vi "Periodic Tasks.vi"(8 "error in":errorcluster) -> ()   [LabVIEW 2019]
doc: "This VI runs in parallel to other tasks. It can contain as many user-defined periodic loops as you need. These can carry out PID or other sorts of timed response."
uses:
  <vilib>/Rock Robotics/WPI/DriverStation/WPI_DriverStationRobotMode2.ctl
  <vilib>/Rock Robotics/WPI/Utilities/WPI_GetSetVariantRefNum.vi
  Robot Global Data.vi
  <vilib>/Rock Robotics/Network Tables/NT Write Boolean.vi
  <vilib>/Rock Robotics/Network Tables/NT Write Number.vi
  <vilib>/Rock Robotics/WPI/RobotDrive/WPI_RobotDriveArcadeDrive_Standard(NoSaturation).vi
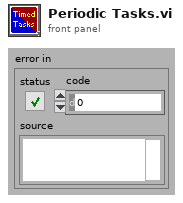
[diagram p1: front panel]
types:
  T1 = typedef "WPI_JoystickDevRef.ctl" = cluster{"Device":T2}
  T2 = typedef "WPI_JoystickDeviceEnum.ctl" = enum16{"USB 0", "USB 1", "USB 2", "USB 3", "USB 4", "USB 5"}
  T3 = typedef "WPI_RobotDriveDevRef.ctl" = cluster{"DevStatus":errorcluster, "Motors[]":T4[], "Square Inputs":bool, "Max Output":dbl}
  T4 = typedef "WPI_MotorControlDeviceRef.ctl" = cluster{"DeviceStatus":errorcluster, "Type":T5, "PWM":cluster{"PWM Channel":T6, "DeadBand":T7}, "CAN":cluster{"Device Number":u8, "SetOutput VI Ref":variant, "GetOutput VI Ref":variant, "Enable VI Ref":variant, "Disable VI Ref":variant, "Data":variant}, "Invert":bool, "DIO PWM":cluster{"PWM \"Enable\" Channel":T6, "DIOChannel":T8, "PWM Rate":dbl}}
  T5 = typedef "WPI_MotorControlType.ctl" = enum16{"PWM", "CAN", "DIO PWM"}
  T6 = typedef "FPGA_DIOPWMChannel.ctl" = enum8{"PWM 0", "PWM 1", "PWM 2", "PWM 3", "PWM 4", "PWM 5", "PWM 6", "PWM 7", "PWM 8", "PWM 9", "PWM MXP 0", "PWM MXP 1", "PWM MXP 2", "PWM MXP 3", "PWM MXP 4", "PWM MXP 5", "PWM MXP 6", "PWM MXP 7", "PWM MXP 8", "PWM MXP 9", "Invalid"}
  T7 = typedef "WPI_PWMDeadband.ctl" = cluster{"Name":string, "maxPositivePwm":i32, "minPositivePwm":i32, "centerPwm":i32, "maxNegativePwm":i32, "minNegativePwm":i32, "angularRange":u16}
  T8 = typedef "FPGA_DIOChannel.ctl" = enum8{"DIO 0", "DIO 1", "DIO 2", "DIO 3", "DIO 4", "DIO 5", "DIO 6", "DIO 7", "DIO 8", "DIO 9", "DIO MXP 0", "DIO MXP 1", "DIO MXP 2", "DIO MXP 3", "DIO MXP 4", "DIO MXP 5", "DIO MXP 6", "DIO MXP 7", "DIO MXP 8", "DIO MXP 9", "DIO MXP 10", "DIO MXP 11", "DIO MXP 12", "DIO MXP 13", "DIO MXP 14", "DIO MXP 15", "SPI Port CS1", "SPI Port CS2", "SPI Port CS3", "SPI Port MISO", "SPI Port MOSI", "Invalid"}
  T9 = cluster{"JoystickDevRef":T1, "RobotDriveDevRef":T3}
  T10 = typedef "WPI_DriverStationRobotMode2.ctl" = enum16{"Autonomous Disabled", "Autonomous Enabled", "Teleop Disabled", "Teleop Enabled", "Disconnected", "Finish", "Test Disabled", "Test Enabled", "Emergency Stopped"}
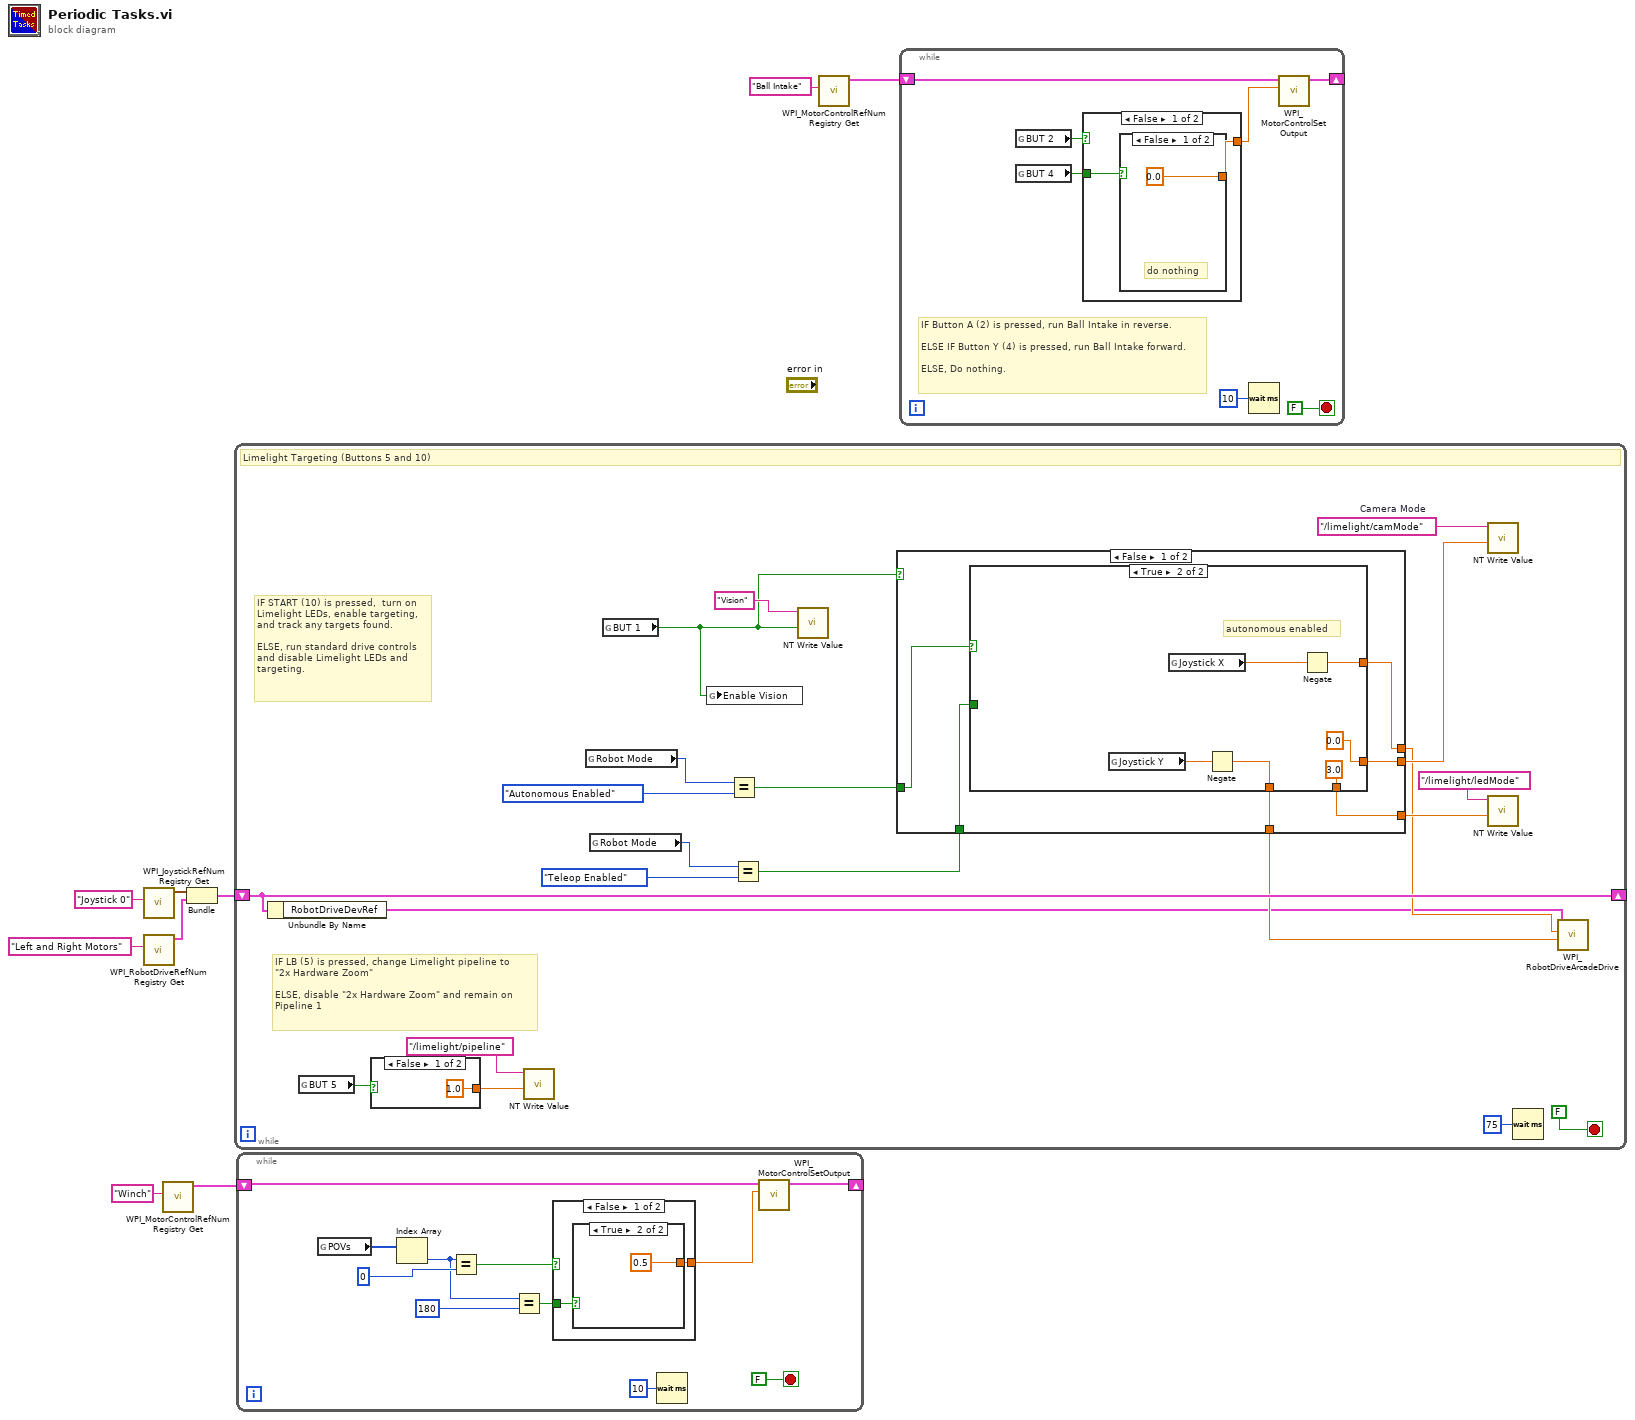
[diagram p0: block diagram]
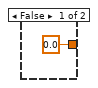
[diagram p2: hidden frame]
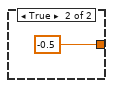
[diagram p3: hidden frame]
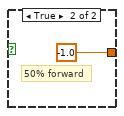
[diagram p4: hidden frame]
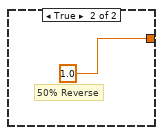
[diagram p5: hidden frame]
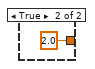
[diagram p6: hidden frame]
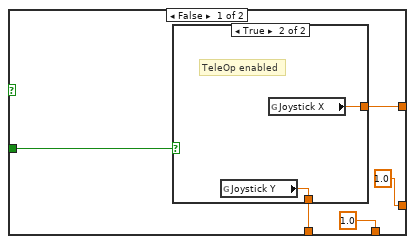
[diagram p7: hidden frame]
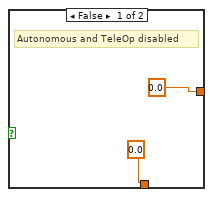
[diagram p8: hidden frame]
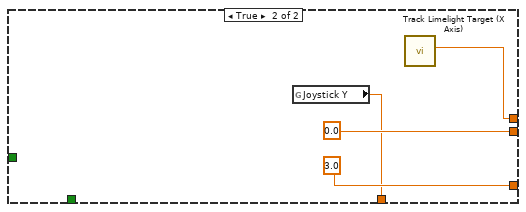
[diagram p9: hidden frame]
diagram:
  n1 = call <vilib>:"WPI_JoystickRefNum Registry Get.vi"("refnum name"="Joystick 0") -> ("JoystickDevRef"=w7:T1)  [unwired: 1 in, 9 out]
  n2 = call <vilib>:"WPI_RobotDriveRefNum Registry Get.vi"("refnum name"="Left and Right Motors") -> ("RobotDriveDevRef"=w6:T3)  [unwired: 1 in, 9 out]
  n3 = call <vilib>:"WPI_MotorControlRefNum Registry Get.vi"("refnum name"="Winch") -> ("MotorControlDevRef"=w2:T4)  [unwired: 9 in, 1 out]
  n4 = Bundle("JoystickDevRef"=w7, "RobotDriveDevRef"=w6) -> (w5:T9)  [unwired: 1 out]
  n5 = while {
    shift-right: [w29] -> _
    shift-left: w5 -> [w29]
    stop <- FALSE stop-if-true
    w27 = "/limelight/camMode"  # Camera Mode
    # "IF LB (5) is pressed, change Limelight pipeline to \n\"2x Hardware Zoom\"\n\nELSE, disable \"2x Hardware Zoom\" and remain on\nPipeline 1"
    # "IF START (10) is pressed,  turn on\nLimelight LEDs, enable targeting,\nand track any targets found.\n\nELSE, run standard drive controls\nand disable Limelight LEDs and \ntargeting."
    # "Limelight Targeting (Buttons 5 and 10)"
    n6 = Unbundle By Name(w29) -> ("RobotDriveDevRef"=w19:T3)
    n7 = global read "Robot Global Data.vi" "BUT 5"() -> (w11:bool)
    n8 = case shown="False" w11 {
      tunnel: [1.0 ("Numeric") 2.0 ("Numeric")] -> w12
      frame False {
      }
      frame True {
      }
    }
    n9 = call-poly <vilib>:"NT Write Value.vi"("Numeric"=w12, "Name"="/limelight/pipeline") -> ()  [unwired: 9 in, 1 out]
    n10 = global read "Robot Global Data.vi" "Robot Mode"() -> (w18:T10)
    n11 = global read "Robot Global Data.vi" "Robot Mode"() -> (w14:T10)
    n12 = global read "Robot Global Data.vi" "BUT 1"() -> (w10:bool)
    n13 = global write "Robot Global Data.vi" "Enable Vision"(w10) -> ()
    n14 = Equal?(x=w18, y=WPI_DriverStationRobotMode2."Autonomous Enabled") -> (x = y?=w16:bool)
    n15 = Equal?(x=w14, y=WPI_DriverStationRobotMode2."Teleop Enabled") -> (x = y?=w13:bool)
    n16 = call-poly <vilib>:"NT Write Value.vi"("Boolean"=w10, "Name"="Vision") -> ()  [unwired: 9 in, 1 out]
    n17 = case shown="False" w10 {
      tunnel: [w34 0.0 ("Numeric")] -> w26
      tunnel: [w33 3.0 ("Numeric")] -> w25
      tunnel: [w37 w55] -> w20
      tunnel: [w38 w54] -> w21
      tunnel: w16 -> [w35 _]
      tunnel: w13 -> [w36 _]
      frame False {
        n18 = case shown="True" w35 {
          tunnel: [w42 w52] -> w38
          tunnel: [w43 w51] -> w37
          tunnel: w36 -> [w41 _]
          tunnel: [1.0 ("Numeric") 0.0 ("Numeric")] -> w34
          tunnel: [1.0 ("Numeric") 3.0 ("Numeric")] -> w33
          frame False {
            n19 = case shown="True" w41 {
              tunnel: [0.0 ("Joystick X") w47] -> w43
              tunnel: [0.0 ("Joystick Y") w46] -> w42
              frame False {
                # "Autonomous and TeleOp disabled"
              }
              frame True {
                # "TeleOp enabled"
                n20 = global read "Robot Global Data.vi" "Joystick Y"() -> (w46:dbl)
                n21 = global read "Robot Global Data.vi" "Joystick X"() -> (w47:dbl)
              }
            }
          }
          frame True {
            # "autonomous enabled"
            n22 = global read "Robot Global Data.vi" "Joystick Y"() -> (w53:dbl)
            n23 = global read "Robot Global Data.vi" "Joystick X"() -> (w50:dbl)
            n24 = Negate(x=w53) -> (-x=w52:dbl)
            n25 = Negate(x=w50) -> (-x=w51:dbl)
          }
        }
      }
      frame True {
        n26 = global read "Robot Global Data.vi" "Joystick Y"() -> (w54:dbl)
        n27 = call "Track Limelight Target (X Axis).vi"() -> ("Joystick X"=w55:dbl)  [unwired: 11 in]
      }
    }
    n28 = call-poly <vilib>:"NT Write Value.vi"("Numeric"=w26, "Name"=w27) -> ()  [unwired: 9 in, 1 out]
    n29 = call-poly <vilib>:"NT Write Value.vi"("Numeric"=w25, "Name"="/limelight/ledMode" ("LED Mode")) -> ()  [unwired: 9 in, 1 out]
    n30 = Wait (ms)(milliseconds to wait=u32 75) -> ()  [unwired: 1 out]
    n31 = call-poly <vilib>:"WPI_RobotDriveArcadeDrive.vi"("Y axis value"=w21, "X axis value"=w20, "RobotDriveDevRef"=w19) -> ()  [unwired: 6 in, 3 out]
  }
  n32 = while {
    shift-right: [w67] -> _
    shift-left: w2 -> [w66]
    stop <- FALSE stop-if-true
    n33 = global read "Robot Global Data.vi" "POVs"() -> (w64:i16[])
    n34 = Index Array(array=w64) -> (element=w60:i16)  [unwired: 1 in]
    n35 = Equal?(x=w60, y=i16 0) -> (x = y?=w63:bool)
    n36 = Equal?(x=w60, y=i16 180) -> (x = y?=w61:bool)
    n37 = case shown="False" w63 {
      tunnel: [w70 -0.5 ("Output")] -> w65
      tunnel: w61 -> [w69 _]
      frame False {
        n38 = case shown="True" w69 {
          tunnel: [0.0 ("Output") 0.5 ("Output")] -> w70
          frame False {
          }
          frame True {
          }
        }
      }
      frame True {
      }
    }
    n39 = Wait (ms)(milliseconds to wait=u32 10) -> ()  [unwired: 1 out]
    n40 = call <vilib>:"WPI_MotorControlSetOutput.vi"("Output"=w65, "MotorControlDevRef"=w66) -> ("MotorControlDevRef"=w67:T4)  [unwired: 7 in, 2 out]
  }
  n41 = call <vilib>:"WPI_MotorControlRefNum Registry Get.vi"("refnum name"="Ball Intake") -> ("MotorControlDevRef"=w3:T4)  [unwired: 9 in, 1 out]
  n42 = while {
    shift-right: [w77] -> _
    shift-left: w3 -> [w78]
    stop <- FALSE stop-if-true
    # "IF Button A (2) is pressed, run Ball Intake in reverse. \n\nELSE IF Button Y (4) is pressed, run Ball Intake forward.\n\nELSE, Do nothing."
    n43 = global read "Robot Global Data.vi" "BUT 2"() -> (w75:bool)
    n44 = global read "Robot Global Data.vi" "BUT 4"() -> (w76:bool)
    n45 = case shown="False" w75 {
      tunnel: [w82 1.0 ("Output")] -> w74
      tunnel: w76 -> [w81 _]
      frame False {
        n46 = case shown="False" w81 {
          tunnel: [0.0 ("Output") -1.0 ("Output")] -> w82
          frame False {
            # "do nothing"
          }
          frame True {
            # "50% forward"
          }
        }
      }
      frame True {
        # "50% Reverse"
      }
    }
    n47 = Wait (ms)(milliseconds to wait=u32 10) -> ()  [unwired: 1 out]
    n48 = call <vilib>:"WPI_MotorControlSetOutput.vi"("Output"=w74, "MotorControlDevRef"=w78) -> ("MotorControlDevRef"=w77:T4)  [unwired: 7 in, 2 out]
  }
